vi "操作GRR表格.vi"(8 "错误输入（无错误）":errorcluster, 9 "数据":string[](array[string]), 10 "位置":string[](array[string]), 11 "路径":path=path "C:/Users/Administrator/Desktop/GRR模板/Test.xlsx") -> (0 "错误输出":errorcluster)   [LabVIEW 2017]
panel:
  in  "数组":enum16{"0", "1", "2"}[](array[ring])
  in  "布尔":bool=TRUE
  in  "Excel._Application 2":refnum<k7>
  in  "枚举":enum16{"0", "1"}(ring)=enum."1"
  in  "Excel._Application":refnum<k7>
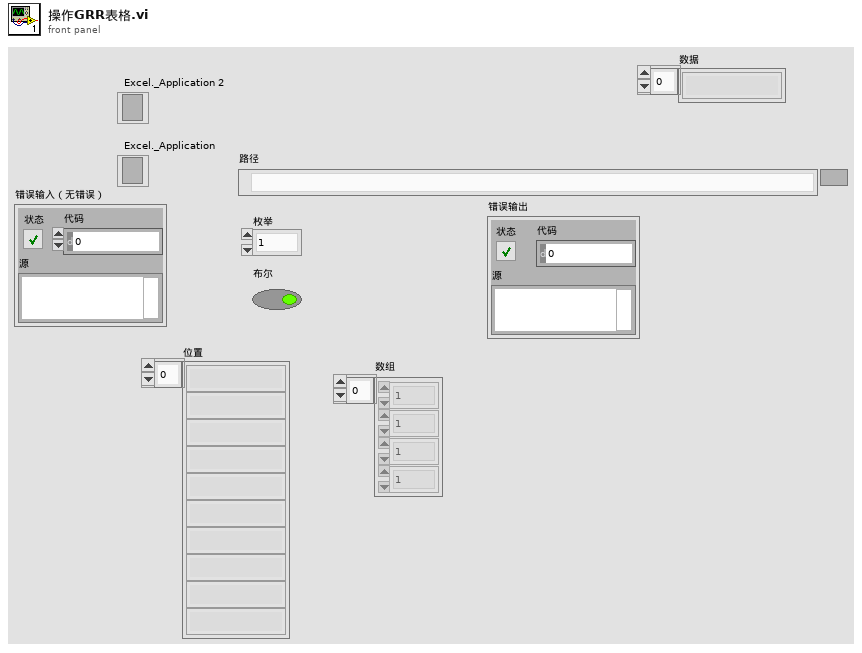
[diagram p1: front panel]
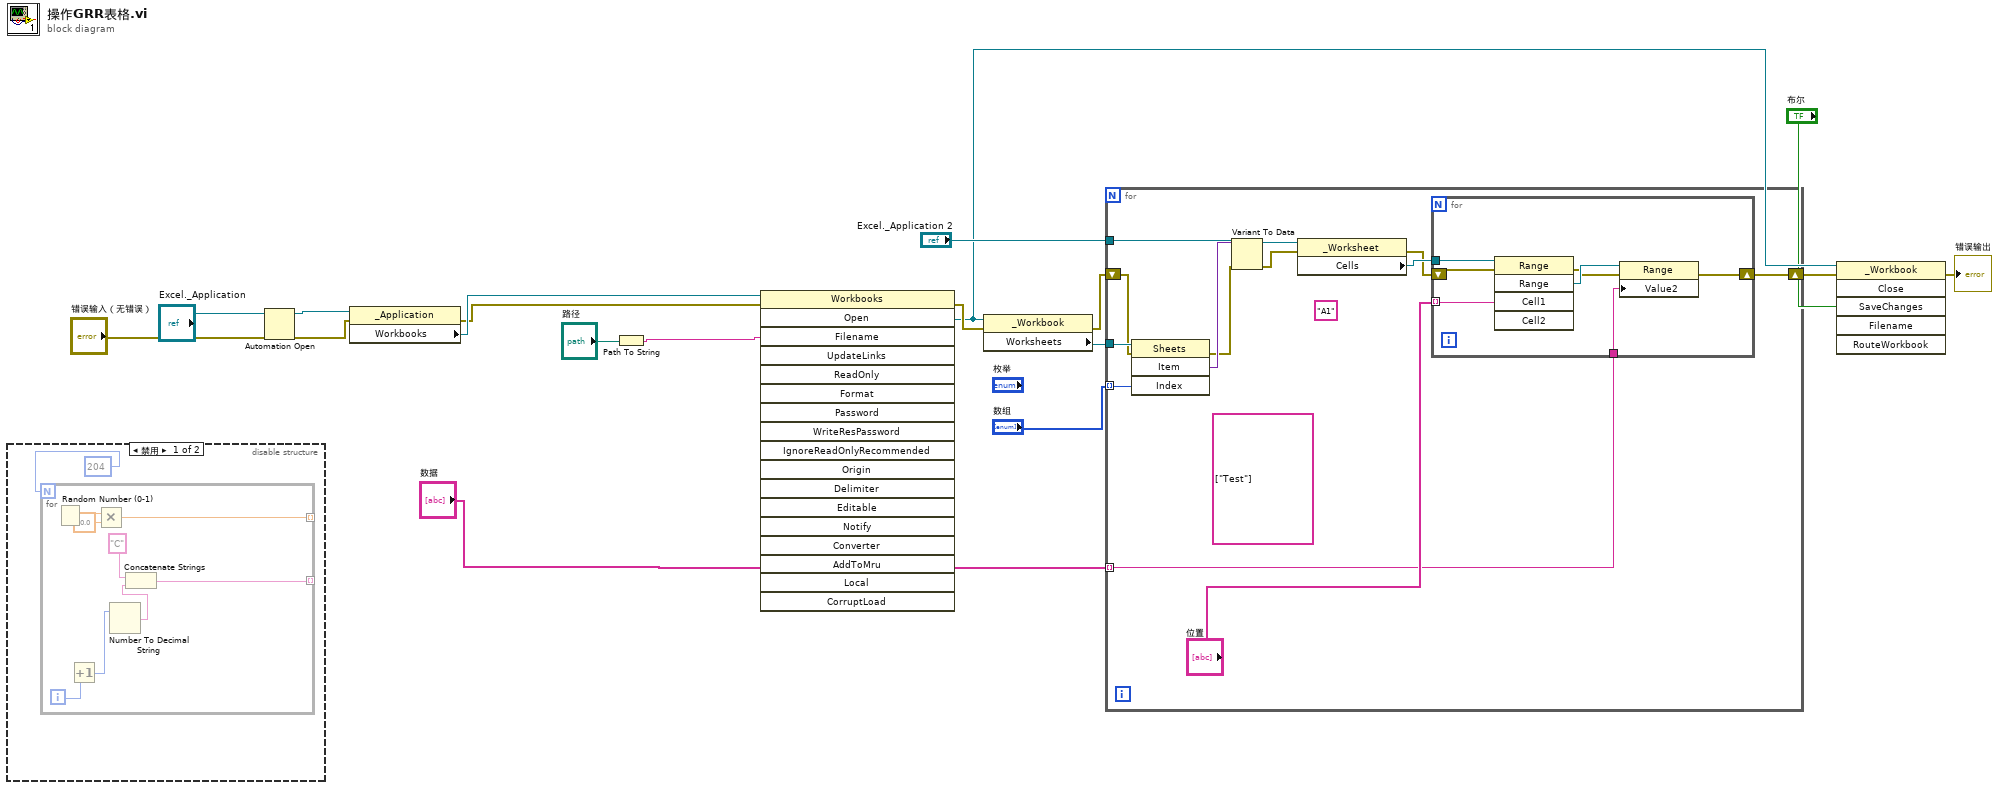
[diagram p0: block diagram]
diagram:
  n1 = disable-structure shown="禁用" {
    frame Disabled {
      n2 = for {
        N: 204 -> [_]
        tunnel: [w25] -> _ mode=indexing
        tunnel: [w20] -> _ mode=indexing
        i -> [w23]
        n3 = Random Number (0-1)() -> (number: 0 to 1=w27:dbl)
        n4 = Increment(x=w23) -> (x+1=w22:i32)
        n5 = Multiply(x=w27, y=10.0) -> (x*y=w25:dbl)
        n6 = Number To Decimal String(number=w22) -> (decimal integer string=w21:string)  [unwired: 1 in]
        n7 = Concatenate Strings("C", w21) -> (w20:string)
      }
    }
    frame Enabled {
    }
  }
  n8 = Automation Open(error in (no error)="错误输入（无错误）", Automation Refnum="Excel._Application") -> (Automation Refnum=w17:refnum<k7>, error out=w4:errorcluster)  [unwired: 2 in]
  n9 = property on="属性节点" class="_Application"(reference=w17, error in=w4) -> (error out=w13:errorcluster, "Workbooks"=w16:refnum<k7>)  [unwired: 1 out]
  n10 = Path To String(path="路径") -> (string=w14:string)
  n11 = invoke on="调用节点" class="Workbooks" method="Open"(reference=w16, error in=w13, "Filename"=w14) -> (error out=w10:errorcluster, "Open"=w8:refnum<k7>)  [unwired: 15 in, 16 out]
  n12 = property on="属性节点" class="_Workbook"(reference=w8, error in=w10) -> (error out=w9:errorcluster, "Worksheets"=w12:refnum<k7>)  [unwired: 1 out]
  n13 = for {
    tunnel: w12 -> [w40]
    tunnel: "数组" -> [w39] mode=indexing
    tunnel: "Excel._Application 2" -> [w37]
    tunnel: "数据" -> [w28] mode=indexing
    shift-right: [w30] -> w7
    shift-left: w9 -> [w34]
    (unwired) string[] ["Test"]
    (unwired) "A1"
    n14 = invoke on="调用节点" class="Sheets" method="Item"(reference=w40, error in=w34, "Index"=w39) -> (error out=w33:errorcluster, "Item"=w38:variant)  [unwired: 1 in, 2 out]
    n15 = Variant To Data(error in=w33, type=w37, Variant=w38) -> (data=w36:refnum<k7>, error out=w32:errorcluster)
    n16 = property on="属性节点" class="_Worksheet"(reference=w36, error in=w32) -> (error out=w31:errorcluster, "Cells"=w35:refnum<k7>)  [unwired: 1 out]
    n17 = for {
      tunnel: w35 -> [w47]
      tunnel: "位置" -> [w46] mode=indexing
      tunnel: w28 -> [w41]
      shift-right: [w42] -> w30
      shift-left: w31 -> [w44]
      n18 = invoke on="调用节点" class="Range" method="Range"(reference=w47, error in=w44, "Cell1"=w46) -> (error out=w43:errorcluster, "Range"=w45:refnum<k7>)  [unwired: 2 in, 3 out]
      n19 = property on="属性节点" class="Range"(reference=w45, error in=w43, "Value2"=w41) -> (error out=w42:errorcluster)  [unwired: 1 out]
    }
  }
  n20 = invoke on="调用节点" class="_Workbook" method="Close"(reference=w8, error in=w7, "SaveChanges"="布尔") -> (error out=→"错误输出":errorcluster)  [unwired: 3 in, 5 out]
